vi "StatuswordToState.vi"(11 "Data_In":u16 format="%.0b") -> (3 "Status":T1)   [LabVIEW 2017, in "WordManipulationLibrary.lvlib"]
uses:
  WordManipulationLibrary.lvlib
  StateMachine.ctl
  Bit Manipulation.lvlib
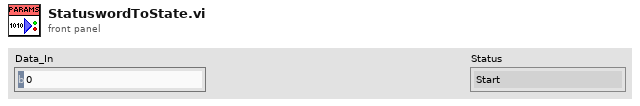
[diagram p1: front panel]
types:
  T1 = typedef "WordManipulationLibrary.lvlib/StateMachine.ctl" = enum16{"Start", "Not Ready to Switch On", "Switch On Disabled", "Ready to Switch On", "Switched On", "Operation enable", "Quick Stop Active", "Fault Reaction Active", "Fault"}
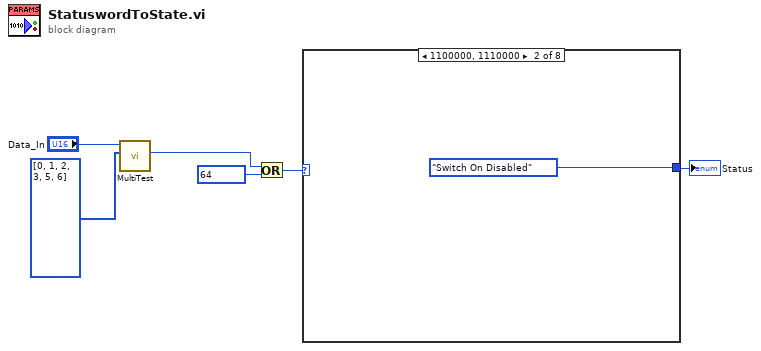
[diagram p0: block diagram]
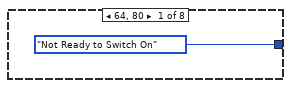
[diagram p2: hidden frame]
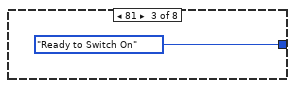
[diagram p3: hidden frame]
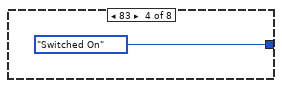
[diagram p4: hidden frame]
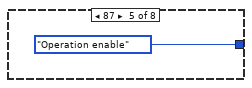
[diagram p5: hidden frame]
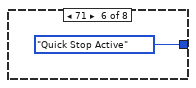
[diagram p6: hidden frame]
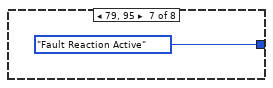
[diagram p7: hidden frame]
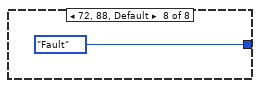
[diagram p8: hidden frame]
diagram:
  n1 = call "MultiTest.vi"("Array"=u8[] [0, 1, 2, 3, 5, 6], "Data_In"="Data_In") -> ("MaskedWord"=w1:u32)  [unwired: 8 in, 1 out]
  n2 = Or(x=w1, y=u32 64) -> (x .or. y?=w5:u32)
  n3 = case shown="1100000, 1110000" w5 {
    tunnel: [StateMachine."Not Ready to Switch On" StateMachine."Switch On Disabled" StateMachine."Ready to Switch On" StateMachine."Switched On" StateMachine."Operation enable" StateMachine."Quick Stop Active" StateMachine."Fault Reaction Active" StateMachine."Fault"] -> w4
    frame 64, 80 {
    }
    frame 96, 112 {
    }
    frame 81 {
    }
    frame 83 {
    }
    frame 87 {
    }
    frame 71 {
    }
    frame 79, 95 {
    }
    frame 72, 88, Default {
    }
  }
  "Status" <- w4
